vi "PH_PP_CurrentMeas.start Task.vi"(0 "i ref in":refnum<vi>, 2 "Task #":i32, 5 "error in (no error)":errorcluster) -> (14 "i ref out":refnum<vi>, 19 "error out":errorcluster)   [LabVIEW 2014, in "PH_PP_CurrentMeas.lvlib"]
uses:
  PH_PP_CurrentMeas.lvlib
  PH_Basics/PH_StatusHandler/PH_StatusHandler.Status.ctl
  PH_Basics/PH_StatusHandler/PH_StatusHandler.lvlib
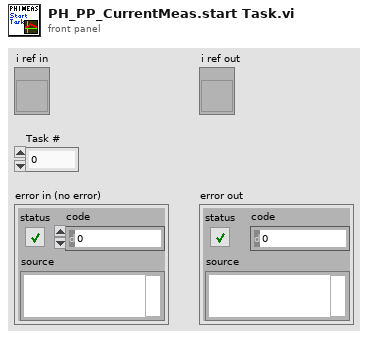
[diagram p1: front panel]
types:
  T1 = typedef "PH_PP_CurrentMeas.lvlib/PH_PP_CurrentMeas.i attribute.ctl" = cluster{"Status":cluster{"GUI Ref Hardware Feedback":refnum<vi>, "Tab Control":refnum<vi>}, "PU 1":cluster{"Instance":string, "Status":T2, "Ref Status ":refnum<vi>, "Data":waveform(dbl)[], "Ref Data":refnum<vi>}, "PU 2":cluster{"Instance":string, "Status":T2, "Ref Status ":refnum<vi>, "Data":waveform(dbl)[], "Ref Data":refnum<vi>}, "PU 3":cluster{"Instance":string, "Status":T2, "Ref Status ":refnum<vi>, "Data":waveform(dbl)[], "Ref Data":refnum<vi>}, "PU 4":cluster{"Instance":string, "Status":T2, "Ref Status ":refnum<vi>, "Data":waveform(dbl)[], "Ref Data":refnum<vi>}, "PU 5":cluster{"Instance":string, "Status":T2, "Ref Status ":refnum<vi>, "Data":waveform(dbl)[], "Ref Data":refnum<vi>}, "FR":cluster{"Instance":string, "Status":T2, "Ref Status ":refnum<vi>, "Data":waveform(dbl)[], "Ref Data":refnum<vi>}, "PA - 19mm 1":cluster{"Instance":string, "Status":T2, "Ref Status ":refnum<vi>}, "PA - 19mm 2":cluster{"Instance":string, "Status":T2, "Ref Status ":refnum<vi>, "no link":bool}, "PA - 45mm":cluster{"Instance":string, "Status":T2, "Ref Status ":refnum<vi>, "no link":bool}, "PA Data":cluster{"Data":waveform(dbl)[], "Ref":refnum<vi>}, "Sequencer":cluster{"Instance":string, "SM State Ref":refnum<vi>}, "Tasks":cluster{"Port":u16, "connection ID":refnum<k5>, "Status":T2, "Ref":refnum<vi>, "Ref Bar":refnum<vi>, "Feedback":cluster{"Received Data Sets":T3[], "Driver Error":errorcluster, "Connection not established":bool, "Error unpacking the data":bool, "No Task defined":bool, "Not triggered yet":bool}, "Data":waveform(dbl)[], "Ref Teststart Task":refnum<vi>}[], "in use":cluster{"MA DP":bool, "FR and PA":bool}, "DAQ Server":string}
  T2 = typedef "PH_StatusHandler.lvlib/PH_StatusHandler.Status.ctl" = i16
  T3 = typedef "PH_PP_CurrentMeas.lvlib/PH_PP_CurrentMeas.CommandCluster.ctl" = cluster{"Command":string, "Data":string, "error out":errorcluster}
  T4 = cluster{"Port":u16, "connection ID":refnum<k5>, "Status":T2, "Ref":refnum<vi>, "Ref Bar":refnum<vi>, "Feedback":cluster{"Received Data Sets":T3[], "Driver Error":errorcluster, "Connection not established":bool, "Error unpacking the data":bool, "No Task defined":bool, "Not triggered yet":bool}, "Data":waveform(dbl)[], "Ref Teststart Task":refnum<vi>}[]
  T5 = cluster{"Port":u16, "connection ID":refnum<k5>, "Status":T2, "Ref":refnum<vi>, "Ref Bar":refnum<vi>, "Feedback":cluster{"Received Data Sets":T3[], "Driver Error":errorcluster, "Connection not established":bool, "Error unpacking the data":bool, "No Task defined":bool, "Not triggered yet":bool}, "Data":waveform(dbl)[], "Ref Teststart Task":refnum<vi>}
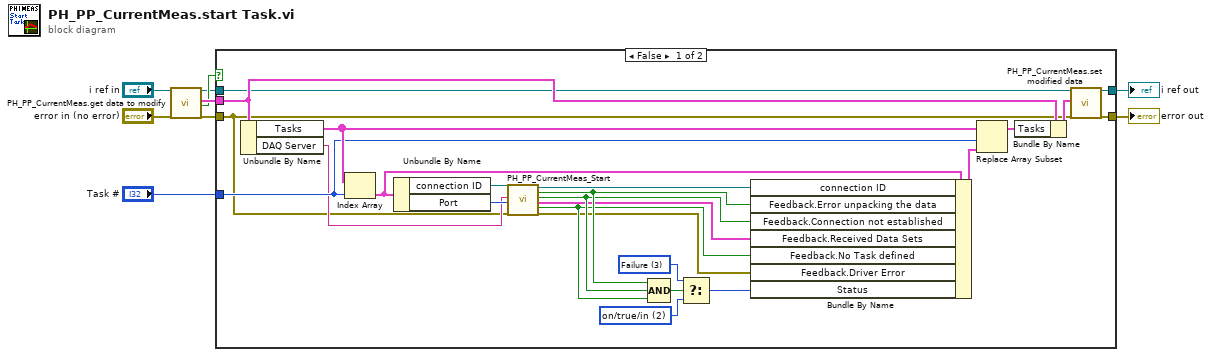
[diagram p0: block diagram]
diagram:
  n1 = call "PH_PP_CurrentMeas.get data to modify.vi"("i ref in"="i ref in", "error in (no error)"="error in (no error)") -> ("i ref out"=w4:refnum<vi>, "i attribute"=w7:T1, "timed out"=w6:bool, "error out"=w5:errorcluster)  [unwired: 14 in]
  n2 = case shown="False" w6 {
    tunnel: w4 -> [w11 w35]
    tunnel: [w33 w35] -> w1
    tunnel: w5 -> [w10 w34]
    tunnel: [w32 w34] -> w2
    tunnel: w7 -> [w13 _]
    tunnel: "Task #" -> [w17 _]
    frame False {
      w25 = T2 2 items=["no info", "off/false/out", "on/true/in", "Failure", "Alarm", "Status 1", "Status 2", "Status 3"] ("f")
      w26 = T2 3 items=["no info", "off/false/out", "on/true/in", "Failure", "Alarm", "Status 1", "Status 2", "Status 3"] ("Status")
      n3 = Unbundle By Name(w13) -> ("Tasks"=w18:T4, "DAQ Server"=w12:string)
      n4 = Index Array(array=w18, index=w17) -> (element=w16:T5)
      n5 = Unbundle By Name(w16) -> ("connection ID"=w15:refnum<k5>, "Port"=w14:u16)
      n6 = call "PH_PP_CurrentMeas_Start.vi"("connection ID in"=w15, "NI6071E DAQ Server"=w12, "Port"=w14, "error in (no error)"=w10) -> ("connection ID out"=w29:refnum<k5>, "Error unpacking the Data?"=w24:bool, "Connection not established"=w23:bool, "Received Data Sets"=w22:T3[], "No Task defined?"=w21:bool, "error out"=w20:errorcluster)  [unwired: 10 in]
      n7 = Compound Arithmetic op=AND(w24, w23, w21) -> (w27:bool)
      n8 = Select(t=w26, s=w27, f=w25) -> (s? t:f=w19:T2)
      n9 = Bundle By Name(cluster=w16, "connection ID"=w29, "Feedback.Error unpacking the data"=w24, "Feedback.Connection not established"=w23, "Feedback.Received Data Sets"=w22, "Feedback.No Task defined"=w21, "Feedback.Driver Error"=w20, "Status"=w19) -> (w28:T5)
      n10 = Replace Array Subset(array=w18, new element=w28, index=w17) -> (w30:T4)
      n11 = Bundle By Name(cluster=w13, "Tasks"=w30) -> (w31:T1)
      n12 = call "PH_PP_CurrentMeas.set modified data.vi"("i ref in"=w11, "i attribute"=w31, "error in (no error)"=w10) -> ("i ref out"=w33:refnum<vi>, "error out"=w32:errorcluster)  [unwired: 15 in]
    }
    frame True {
    }
  }
  "error out" <- w2
  "i ref out" <- w1
